vi "Loop Till Force Sensed.vi"() -> ()   [LabVIEW 2013]
uses:
  <vilib>/Analysis/baseanly.llb/Mean (DBL).vi
  <vilib>/LabVIEW Interface for Arduino/LabVIEW Interface for Arduino.lvlib
  <vilib>/Analysis/NI_AALBase.lvlib
panel:
  out "Force Threshhold Reached":bool
  out "Force Average":dbl format="%0.2f"
  out "Force vs Time":dbl[](graph)
  out "Voltage Average":dbl format="%0.2f"
  in  "Array":dbl[](array[numeric])
  in  "Sample Rate (HZ)":u16
  in  "Analog Input Pin":u8
  in  "Stop":bool
  out "Volatege vs Time":dbl[](graph)
  out "output array":dbl[](array[numeric])
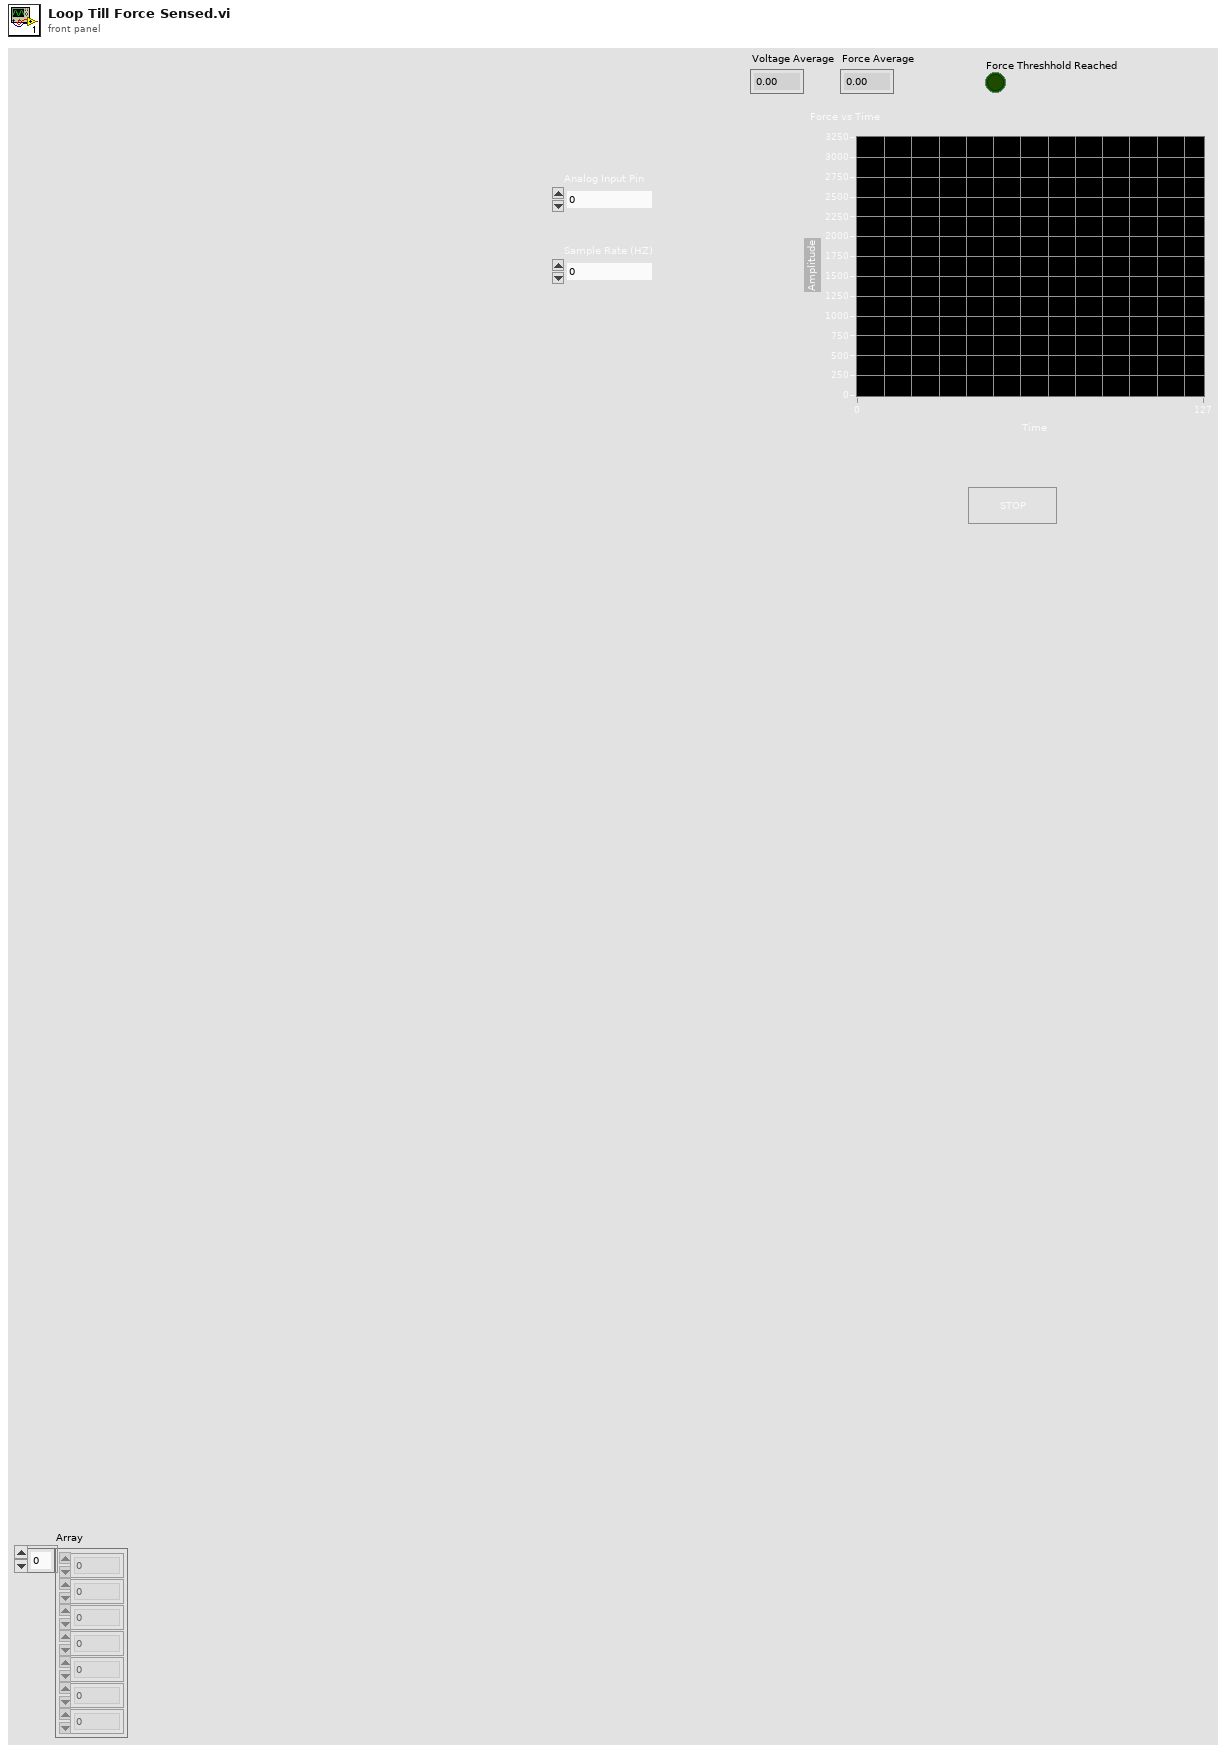
[diagram p1: front panel]
types:
  T1 = typedef "LabVIEW Interface for Arduino.lvlib/Arduino Resource.ctl" = cluster{"VISA resource":refnum<visa-resource-name>, "Board Type":T2, "Connection Type":enum8{"USB / Serial"}, "Bytes Per Packet (15)":u8}
  T2 = typedef "LabVIEW Interface for Arduino.lvlib/Board Type.ctl" = enum16{"Uno", "Dimuelanove w/Atmega 328", "Mega 2560"}
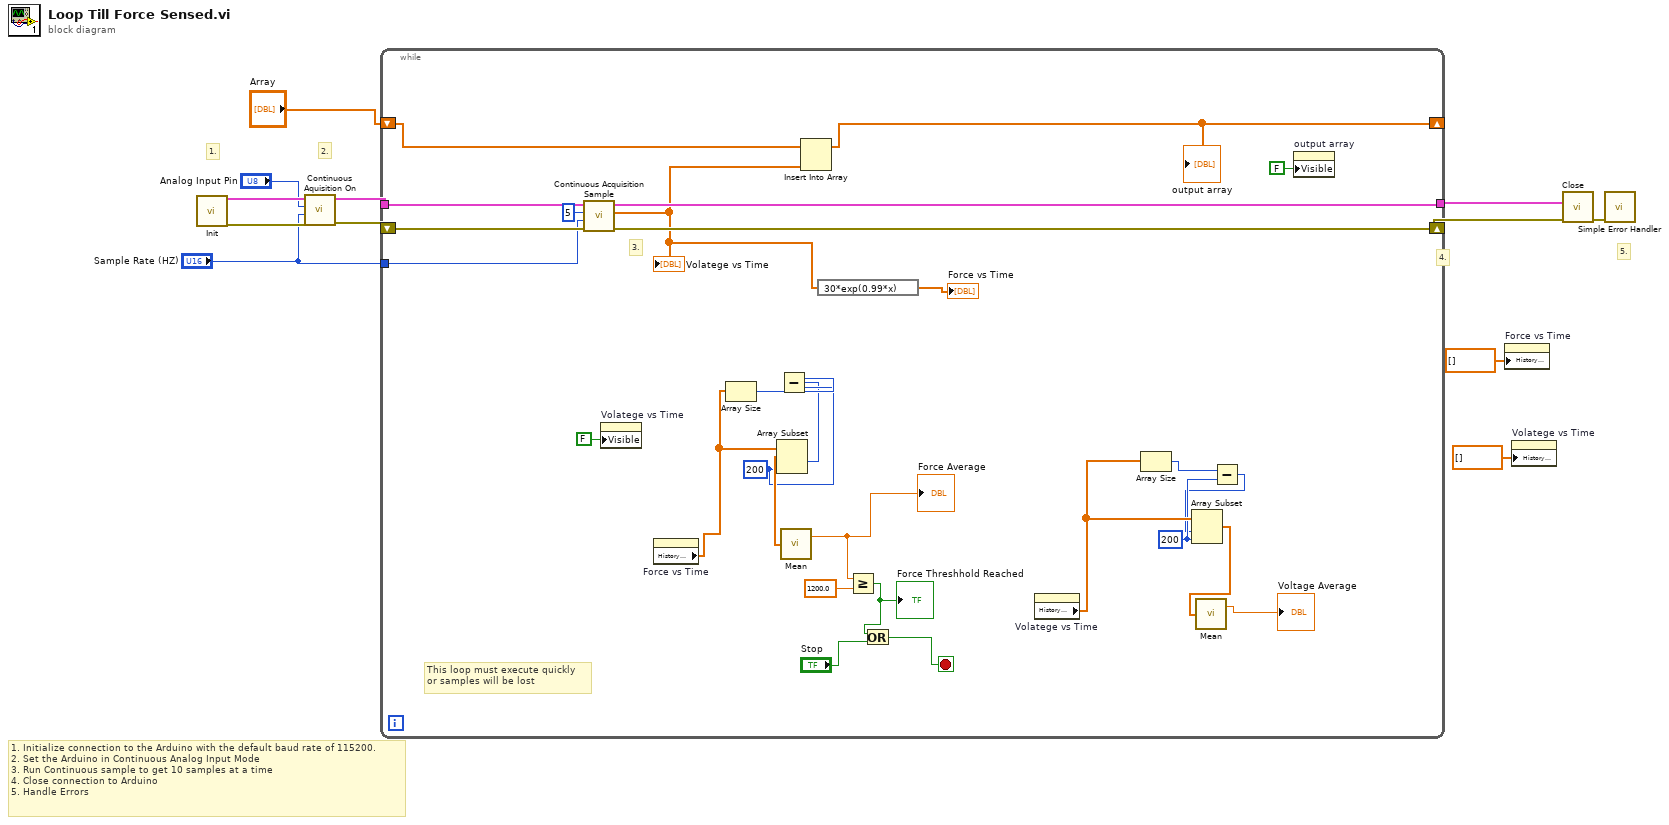
[diagram p0: block diagram]
diagram:
  # "5."
  # "4."
  # "2."
  # "1."
  # "1. Initialize connection to the Arduino with the default baud rate of 115200.\n2. Set the Arduino in Continuous Analog Input Mode\n3. Run Continuous sample to get 10 samples at a time\n4. Close connection to Arduino\n5. Handle Errors"
  n1 = call <vilib>:"Init.vi"() -> ("Arduino Resource"=w12:T1, "error out"=w5:errorcluster)  [unwired: 18 in]
  n2 = call <vilib>:"Continuous Aquisition On.vi"("error in"=w5, "Acquition Speed"="Sample Rate (HZ)", "Analog Input Pin"="Analog Input Pin", "Arduino Resource"=w12) -> ("error out"=w10:errorcluster, "Arduino Resource"=w11:T1)  [unwired: 6 in]
  n3 = while {
    tunnel: w11 -> [w40]
    tunnel: [w39] -> w9
    shift-right: [w38] -> w6
    shift-left: w10 -> [w37]
    tunnel: "Sample Rate (HZ)" -> [w35]
    shift-right: [w33] -> _
    shift-left: "Array" -> [w34]
    stop <- w15 stop-if-true
    w24 = 200 ("length")
    w21 = 200 ("length")
    # "This loop must execute quickly\nor samples will be lost"
    # "3."
    n4 = call <vilib>:"Continuous Acquisition Sample.vi"("Arduino Resource"=w40, "Samples to Read"=u16 5, "Sample Rate (HZ)"=w35, "error in (no error)"=w37) -> ("Arduino Resource"=w39:T1, "Data"=w32:dbl[], "error out"=w38:errorcluster)  [unwired: 4 in]
    "Volatege vs Time" <- w32
    n5 = property on="Volatege vs Time" class="WFChart (strict)"("Visible"=FALSE) -> ()  [unwired: 2 in, 2 out]
    n6 = property on="Force vs Time" class="WFChart (strict)"() -> ("History Data"=w30:dbl[])  [unwired: 2 in, 2 out]
    n7 = Array Size(array=w30) -> (size(s)=w22:i32)
    n8 = Subtract(x=w22, y=w21) -> (x-y=w20:i32)
    n9 = Array Subset(array=w30, index=w20, length=w21) -> (w29:dbl[])
    n10 = call-poly <vilib>:"Mean.vi"("X"=w29) -> ("mean"=w19:dbl)  [unwired: 1 out]
    "Force Average" <- w19
    n11 = Insert Into Array(array=w34, new element=w32) -> (w33:dbl[])  [unwired: 1 in]
    "output array" <- w33
    n12 = expression code="30*exp(0.99*x)"(w32) -> (→"Force vs Time":dbl[])
    n13 = Greater Or Equal?(x=w19, y=1200.0) -> (x >= y?=w17:bool)
    "Force Threshhold Reached" <- w17
    n14 = Or(x=w17, y="Stop") -> (x .or. y?=w15:bool)
    n15 = property on="Volatege vs Time" class="WFChart (strict)"() -> ("History Data"=w28:dbl[])  [unwired: 2 in, 2 out]
    n16 = Array Size(array=w28) -> (size(s)=w25:i32)
    n17 = Subtract(x=w25, y=w24) -> (x-y=w23:i32)
    n18 = Array Subset(array=w28, index=w23, length=w24) -> (w26:dbl[])
    n19 = call-poly <vilib>:"Mean.vi"("X"=w26) -> ("mean"=→"Voltage Average":dbl)  [unwired: 1 out]
    n20 = property on="output array" class="Arr (strict)"("Visible"=FALSE) -> ()  [unwired: 2 in, 2 out]
  }
  n21 = property on="Force vs Time" class="WFChart (strict)"("History Data"=dbl[] []) -> ()  [unwired: 2 in, 2 out]
  n22 = property on="Volatege vs Time" class="WFChart (strict)"("History Data"=dbl[] []) -> ()  [unwired: 2 in, 2 out]
  n23 = call <vilib>:"Close.vi"("Arduino Resource"=w9, "error in"=w6) -> ("error out"=w8:errorcluster)  [unwired: 13 in]
  n24 = call <vilib>:"Simple Error Handler.vi"("error in (no error)"=w8) -> ()  [unwired: 4 in, 5 out]
